vi "Enqueue Blocks.vi"(10 "data":u8[](array[numeric]), 11 "Blocks queue":refnum<queue>) -> ()   [LabVIEW 2013, in "SHA-1.lvlib" / "SHA-1.lvclass"]
uses:
  SHA-1.lvclass
  Data-vector.ctl
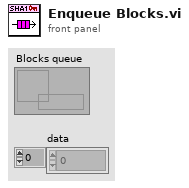
[diagram p1: front panel]
types:
  T1 = typedef "SHA-1.lvlib/SHA-1.lvclass/Data-vector.ctl" = cluster{"Data[ ]":u8[], "end":bool}
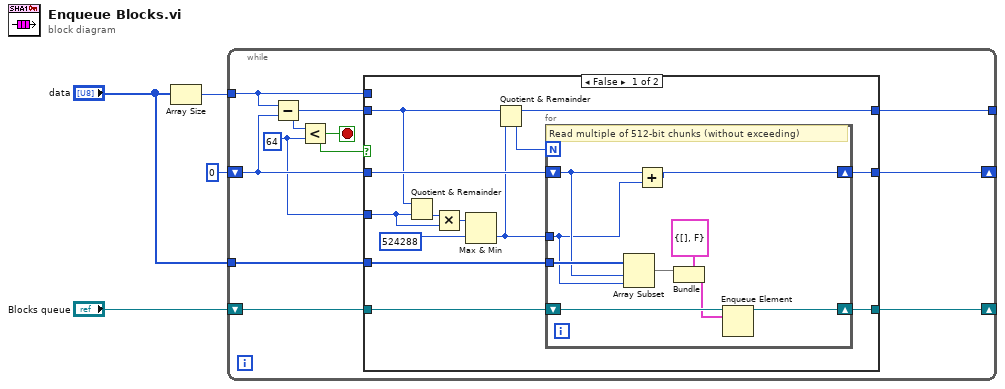
[diagram p0: block diagram]
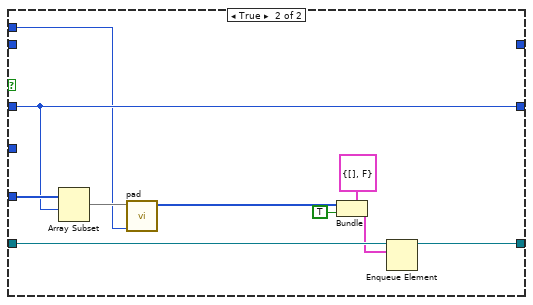
[diagram p2: hidden frame]
diagram:
  n1 = Array Size(array="data") -> (size(s)=w4:i32)
  n2 = while {
    shift-right: [w10] -> _
    shift-left: 0 -> [w12]
    tunnel: w4 -> [w5]
    tunnel: [w11] -> _
    tunnel: "data" -> [w9]
    shift-right: [w13] -> _
    shift-left: "Blocks queue" -> [w14]
    stop <- w6 stop-if-true
    w7 = 64 ("y")
    n3 = Subtract(x=w5, y=w12) -> (x-y=w8:i32)
    n4 = Less?(x=w8, y=w7) -> (x < y?=w6:bool)
    n5 = case shown="False" w6 {
      tunnel: w14 -> [w27 w44]
      tunnel: [w26 w43] -> w13
      tunnel: w12 -> [w25 w45]
      tunnel: [w19 _] -> w11
      tunnel: [w18 w45] -> w10
      tunnel: w9 -> [w17 w46]
      tunnel: w8 -> [w16 _]
      tunnel: w7 -> [w15 _]
      tunnel: w5 -> [_ w38]
      frame False {
        n6 = Quotient & Remainder(x=w16, y=w15) -> (floor(x/y)=w24:i32)  [unwired: 1 out]
        n7 = Multiply(x=w24, y=w15) -> (x*y=w23:i32)
        n8 = Max & Min(x=w23, y=524288) -> (min(x,y)=w20:i32)  [unwired: 1 out]
        n9 = Quotient & Remainder(x=w16, y=w20) -> (x-y*floor(x/y)=w19:i32, floor(x/y)=w21:i32)
        n10 = for {
          N: w21 -> [_]
          shift-right: [w35] -> w26
          shift-left: w27 -> [w36]
          shift-right: [w29] -> w18
          shift-left: w25 -> [w31]
          tunnel: w20 -> [w30]
          tunnel: w17 -> [w33]
          # "Read multiple of 512-bit chunks (without exceeding)"
          n11 = Array Subset(array=w33, index=w31, length=w30) -> (w32:u8[])
          n12 = Add(x=w31, y=w30) -> (x+y=w29:i32)
          n13 = Bundle(cluster=T1 {"Data[ ]"=[], "end"=FALSE}, "Data[ ]"=w32) -> (w34:T1)  [unwired: 1 in]
          n14 = Enqueue Element(queue=w36, element=w34) -> (queue out=w35:refnum<queue>)  [unwired: 2 in, 2 out]
        }
      }
      frame True {
        n15 = Array Subset(array=w46, index=w45) -> (w39:u8[])  [unwired: 1 in]
        n16 = call "pad.vi"("data length"=w38, "Last Block"=w39) -> ("Padding"=w37:u8[])  [unwired: 8 in, 1 out]
        n17 = Bundle(cluster=T1 {"Data[ ]"=[], "end"=FALSE}, "Data[ ]"=w37, "end"=TRUE) -> (w41:T1)
        n18 = Enqueue Element(queue=w44, element=w41) -> (queue out=w43:refnum<queue>)  [unwired: 2 in, 2 out]
      }
    }
  }
